vi "Start Async.vi"(8 "error in (no error)":errorcluster, 11 "gRPC Server in":refnum<class "Manager.lvclass">) -> (0 "error out":errorcluster, 3 "gRPC Server out":refnum<class "Manager.lvclass">)   [LabVIEW 2021, in "CIF_Manager_server.lvlib" / "Manager.lvclass"]
uses:
  Manager.lvclass
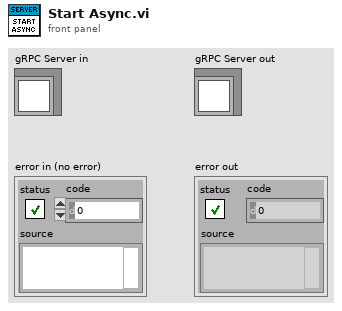
[diagram p1: front panel]
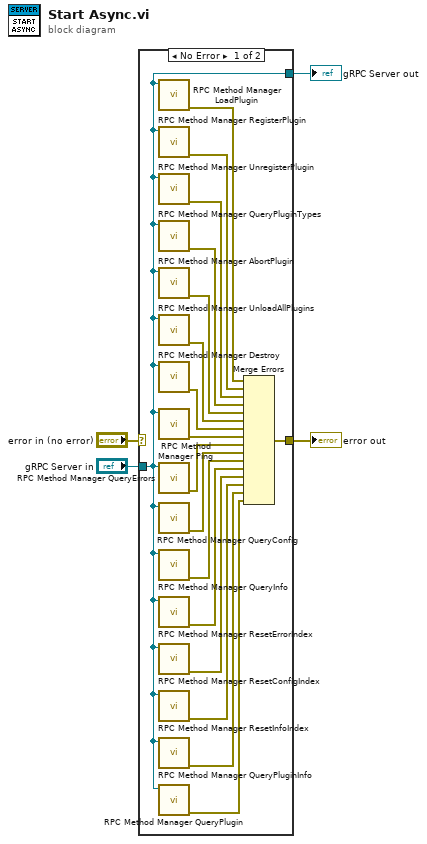
[diagram p0: block diagram]
diagram:
  n1 = case shown="No Error" "error in (no error)" {
    selector: "error in (no error)" -> [_ w24]
    tunnel: [w22 w24] -> w3
    tunnel: [w21 w23] -> w1
    tunnel: "gRPC Server in" -> [w21 w23]
    frame No Error {
      n2 = call "RPC Method Manager LoadPlugin.vi"("OOP Server in"=w21) -> ("error out"=w20:errorcluster)  [unwired: 9 in, 1 out]
      n3 = call "RPC Method Manager RegisterPlugin.vi"("OOP Server in"=w21) -> ("error out"=w19:errorcluster)  [unwired: 9 in, 1 out]
      n4 = call "RPC Method Manager UnregisterPlugin.vi"("OOP Server in"=w21) -> ("error out"=w18:errorcluster)  [unwired: 9 in, 1 out]
      n5 = call "RPC Method Manager QueryPluginTypes.vi"("OOP Server in"=w21) -> ("error out"=w17:errorcluster)  [unwired: 9 in, 1 out]
      n6 = call "RPC Method Manager AbortPlugin.vi"("OOP Server in"=w21) -> ("error out"=w16:errorcluster)  [unwired: 9 in, 1 out]
      n7 = call "RPC Method Manager UnloadAllPlugins.vi"("OOP Server in"=w21) -> ("error out"=w15:errorcluster)  [unwired: 9 in, 1 out]
      n8 = call "RPC Method Manager Destroy.vi"("OOP Server in"=w21) -> ("error out"=w14:errorcluster)  [unwired: 9 in, 1 out]
      n9 = call "RPC Method Manager Ping.vi"("OOP Server in"=w21) -> ("error out"=w13:errorcluster)  [unwired: 9 in, 1 out]
      n10 = call "RPC Method Manager QueryErrors.vi"("OOP Server in"=w21) -> ("error out"=w12:errorcluster)  [unwired: 9 in, 1 out]
      n11 = call "RPC Method Manager QueryConfig.vi"("OOP Server in"=w21) -> ("error out"=w11:errorcluster)  [unwired: 9 in, 1 out]
      n12 = call "RPC Method Manager QueryInfo.vi"("OOP Server in"=w21) -> ("error out"=w10:errorcluster)  [unwired: 9 in, 1 out]
      n13 = call "RPC Method Manager ResetErrorIndex.vi"("OOP Server in"=w21) -> ("error out"=w9:errorcluster)  [unwired: 9 in, 1 out]
      n14 = call "RPC Method Manager ResetConfigIndex.vi"("OOP Server in"=w21) -> ("error out"=w8:errorcluster)  [unwired: 9 in, 1 out]
      n15 = call "RPC Method Manager ResetInfoIndex.vi"("OOP Server in"=w21) -> ("error out"=w7:errorcluster)  [unwired: 9 in, 1 out]
      n16 = call "RPC Method Manager QueryPluginInfo.vi"("OOP Server in"=w21) -> ("error out"=w6:errorcluster)  [unwired: 9 in, 1 out]
      n17 = call "RPC Method Manager QueryPlugin.vi"("OOP Server in"=w21) -> ("error out"=w5:errorcluster)  [unwired: 9 in, 1 out]
      n18 = Merge Errors(w20, w19, w18, w17, w16, w15, w14, w13, w12, w11, w10, w9, w8, w7, w6, w5) -> (w22:errorcluster)
    }
    frame Error {
    }
  }
  "error out" <- w3
  "gRPC Server out" <- w1
